vi "Pre Launch Init.vi"(11 "IED in":refnum<class "IED.lvclass">) -> (0 "error out":errorcluster, 3 "IED out":refnum<class "IED.lvclass">)   [LabVIEW 2015, in "IED Actor.lvlib" / "IED.lvclass"]
doc: "(<B>Filename</B>: Actor Framework.lvlib:Actor.lvclass:Pre Launch Init.vi)\n\nDefines behavior that occurs after the Launch Nested Actor method is invoked but before the actor's Actor Core method begins running.\n\nBy default, this method does nothing. A descendant class may override it to define behavior."
uses:
  IED.lvclass
  IED.lvclass/IED.ctl
  <vilib>/ActorFramework/Actor/Actor.lvclass
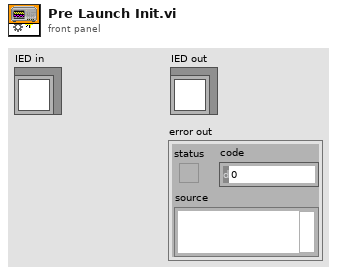
[diagram p1: front panel]
types:
  T1 = typedef "IED Actor.lvlib/IED.lvclass/Notifiers Cluster.ctl" = cluster{"stop":refnum<notifier>, "stop check":refnum<notifier>, "stop watchdog":refnum<notifier>, "IED stop":refnum<notifier>, "Island stop":refnum<notifier>, "Dog stop":refnum<notifier>}
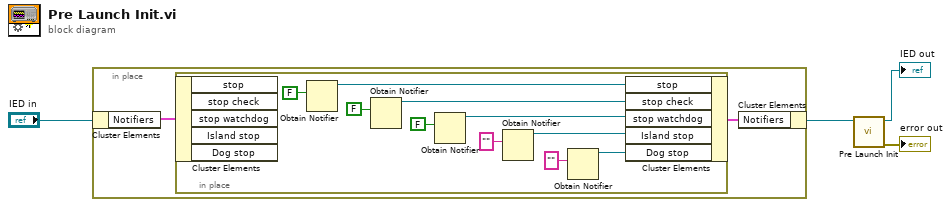
[diagram p0: block diagram]
diagram:
  n1 = in-place {
    n2 = in-place-cluster #1("IED in") -> ("Notifiers"=w6:T1)
    n3 = in-place {
      n4 = in-place-cluster #2(w6) -> ()  [unwired: 5 out]
      n5 = Obtain Notifier(notification data type=FALSE) -> (notifier out=w15:refnum<notifier>)  [unwired: 3 in, 2 out]
      n6 = Obtain Notifier(notification data type=FALSE) -> (notifier out=w14:refnum<notifier>)  [unwired: 3 in, 2 out]
      n7 = Obtain Notifier(notification data type=FALSE) -> (notifier out=w12:refnum<notifier>)  [unwired: 3 in, 2 out]
      n8 = Obtain Notifier(notification data type="" ("name (unnamed)")) -> (notifier out=w10:refnum<notifier>)  [unwired: 3 in, 2 out]
      n9 = Obtain Notifier(notification data type="" ("name (unnamed)")) -> (notifier out=w7:refnum<notifier>)  [unwired: 3 in, 2 out]
      n10 = in-place-cluster #2("stop"=w15, "stop check"=w14, "stop watchdog"=w12, "Island stop"=w10, "Dog stop"=w7) -> (w5:T1)
    }
    n11 = in-place-cluster #1("Notifiers"=w5) -> (w1:refnum<class "IED.lvclass">)
  }
  n12 = call-parent "Pre Launch Init.vi"("Actor in"=w1) -> ("error out"=→"error out":errorcluster, "Actor out"=→"IED out":refnum<class "IED.lvclass">)  [unwired: 9 in]
